vi "DAQmx Create Channel (AI-Position-EddyCurrentProxProbe).vi"(0 "task in":refnum<k21>, 1 "maximum value":dbl=0.00254 format="%.5f", 2 "minimum value":dbl format="%0.2f", 5 "physical channels":tag, 7 "name to assign":string, 9 "units":i32(ring)=10219 items=["Meters"=10219, "Inches"=10379, "From Custom Scale"=10065], 11 "error in":errorcluster, 12 "custom scale name":tag, 13 "sensitivity":dbl=200.0, 14 "sensitivity units":i32(ring)=14836 items=["mVolts/mil"=14836, "Volts/mil"=14837, "mVolts/mm"=14838, "Volts/mm"=14839, "mVolts/micron"=14840]) -> (4 "task out":refnum<k21>, 15 "error out":errorcluster)   [LabVIEW 2011]
doc: "Creates channel(s) that use an eddy current proximity probe to measure position."
uses:
  C:/Program Files/National Instruments/LabVIEW 2011/resource/objmgr/daqmx.rc
panel:
  # "input limits"
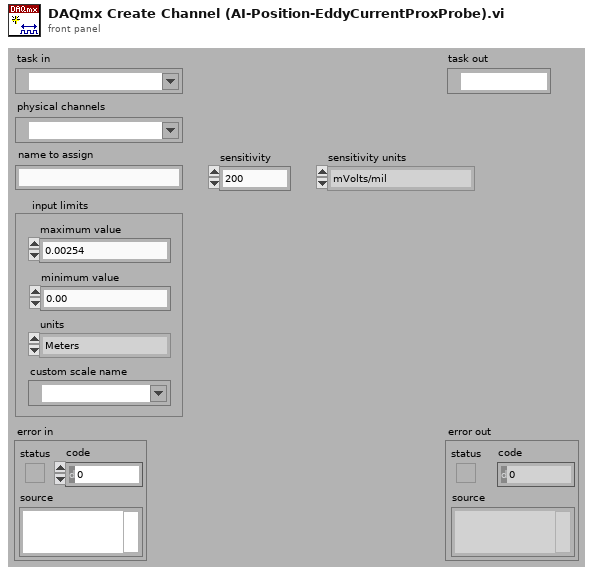
[diagram p1: front panel]
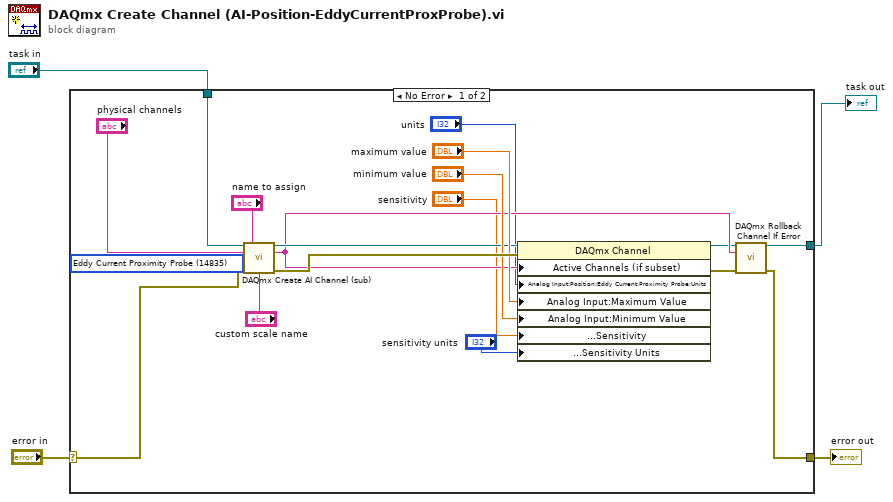
[diagram p0: block diagram]
diagram:
  n1 = case shown="No Error" "error in" {
    selector: "error in" -> [w21 w24]
    tunnel: [w12 w24] -> w2
    tunnel: "task in" -> [w22 w23]
    tunnel: [w13 w23] -> w1
    frame No Error {
      w6 = 14835 items=["Voltage"=10322, "Current"=10134, "More:Voltage:Custom with Excitation"=10323, "More:Current:Custom with Excitation"=10136, "Frequency"=10181, "Period"=10257, "Resistance"=10278, "Temperature:Thermocouple"=10303, "Temperature:Thermistor"=10302, "Temperature:RTD"=10301, "Temperature:Built-in Sensor"=10311, "Strain Gage"=10300, "LVDT"=10352, "RVDT"=10353, "Accelerometer:Voltage Input"=10355, "Accelerometer:Current Input"=10356, "Eddy Current Proximity Probe"=14835] ("measurement type")
      n2 = call "DAQmx Create AI Channel (sub).vi"("task in"=w22, "virtual channel name"="name to assign", "physical channel name"="physical channels", "measurement type"=w6, "error in"=w21, "custom scale"="custom scale name") -> ("task out"=w14:refnum<k21>, "channel names"=w11:string, "error out"=w18:errorcluster)  [unwired: 1 in, 6 out]
      n3 = property class="DAQmx Channel"(reference=w14, error in=w18, "Active Channels (if subset)"=w11, "Analog Input:Position:Eddy Current Proximity Probe:Units"="units", "Analog Input:Maximum Value"="maximum value", "Analog Input:Minimum Value"="minimum value", "Analog Input:Position:Eddy Current Proximity Probe:Sensitivity"="sensitivity", "Analog Input:Position:Eddy Current Proximity Probe:Sensitivity Units"="sensitivity units") -> (reference out=w10:refnum<k21>, error out=w9:errorcluster)
      n4 = call "DAQmx Rollback Channel If Error.vi"("task in"=w10, "channel names"=w11, "error in"=w9) -> ("task out"=w13:refnum<k21>, "error out"=w12:errorcluster)  [unwired: 11 out]
    }
    frame Error {
    }
  }
  "error out" <- w2
  "task out" <- w1
